vi "ma_FFT Power Spectrum and PS Density no State.vi"(0 "time signal":waveform(dbl), 1 "restart averaging (F)":bool, 2 "ps density":bool, 5 "window":T1=1 items=["Rectangle"=0, "Hanning"=1, "Hamming"=2, "Blackman-Harris"=3, "Exact Blackman"=4, "Blackman"=5, "Flat Top"=6, "4 Term B-Harris "=7, "7 Term B-Harris"=8, "Low Sidelobe"=9, "Blackman Nuttall"=11, "Triangle"=30, "Bartlett-Hanning"=31, "Bohman"=32, "Parzen"=33, "Welch"=34, "Kaiser"=60, "Dolph-Chebyshev"=61, "Gaussian"=62], 7 "averaging parameters":T3={"averaging mode"=enum."No averaging", "weighting mode"=enum."Exponential", "number of averages"=10} {"number of averages" min=1}, 9 "dB On (F)":bool, 11 "error in":errorcluster, 12 "state info":T2 {"real spectrum" format="%0.2f"; "averages completed" format="%0.2f"; "df" format="%0.2f"; "complex spectrum" format="%0.2f"; "spectrum parameters"."window" items=["Rectangle"=0, "Hanning"=1, "Hamming"=2, "Blackman-Harris"=3, "Exact Blackman"=4, "Blackman"=5, "Flat Top"=6, "4 Term B-Harris "=7, "7 Term B-Harris"=8, "Low Sidelobe"=9, "Blackman Nuttall"=11, "Triangle"=30, "Bartlett-Hanning"=31, "Bohman"=32, "Parzen"=33, "Welch"=34, "Kaiser"=60, "Dolph-Chebyshev"=61, "Gaussian"=62]; "dt" format="%0.2f"; "timestamp" format="%0.2f"; "dt history" format="%0.2f"; "t0 history" format="%0.2f"}, 13 "window parameter":dbl=nan) -> (3 "averaging done":bool, 4 "power spectrum":cluster{"f0":dbl, "df":dbl, "magnitude":dbl[]} {"f0" format="%0.2p"; "df" format="%0.2p"; "magnitude" format="%0.2p"}, 10 "averages completed":dbl format="%0.2f", 14 "state info":T2 {"real spectrum" format="%0.2f"; "averages completed" format="%0.2f"; "df" format="%0.2f"; "complex spectrum" format="%0.2f"; "spectrum parameters"."window" items=["Rectangle"=0, "Hanning"=1, "Hamming"=2, "Blackman-Harris"=3, "Exact Blackman"=4, "Blackman"=5, "Flat Top"=6, "4 Term B-Harris "=7, "7 Term B-Harris"=8, "Low Sidelobe"=9, "Blackman Nuttall"=11, "Triangle"=30, "Bartlett-Hanning"=31, "Bohman"=32, "Parzen"=33, "Welch"=34, "Kaiser"=60, "Dolph-Chebyshev"=61, "Gaussian"=62]; "dt" format="%0.2f"; "timestamp" format="%0.2f"; "dt history" format="%0.2f"; "t0 history" format="%0.2f"}, 15 "error out":errorcluster)   [LabVIEW 2020, in "NI_MAPro.lvlib"]
doc: "Computes the averaged auto power spectrum of the input signal. Each time waveform corresponds to a single FFT block and has to be passed individually to this VI. Averaging parameters specifies how the averaging is performed. This includes the averaging mode (No averaging, vector averaging, RMS averaging, or peak hold), the weighting mode (linear or exponential), and the number of averages. Averages completed returns the number of averages completed so far."
uses:
  NI_MAPro.lvlib
  windowTd.ctl
  NI_MABase.lvlib
  NI_AALPro.lvlib
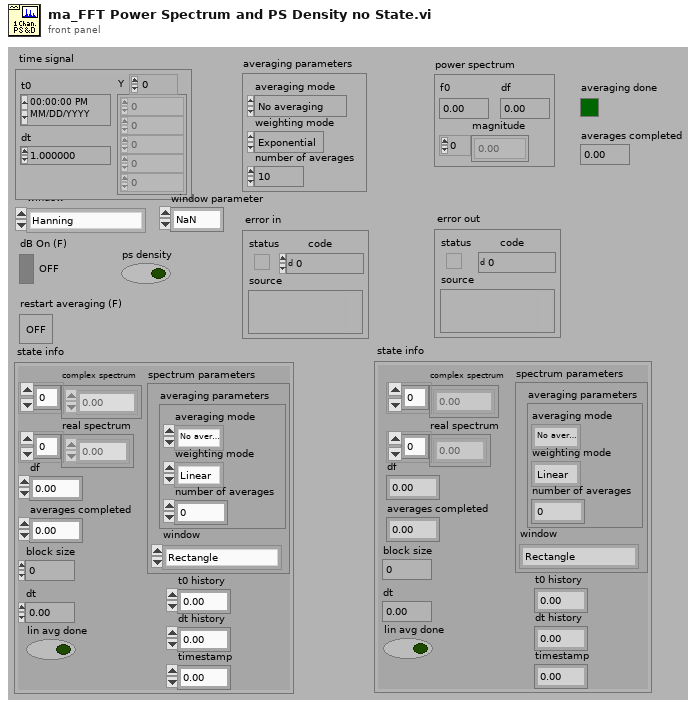
[diagram p1: front panel]
types:
  T1 = typedef "NI_AALPro.lvlib/windowTd.ctl" = u32
  T2 = cluster{"block size":i32, "dt":dbl, "spectrum parameters":cluster{"averaging parameters":cluster{"averaging mode":enum16{"No averaging", "Vector averaging", "RMS averaging", "Peak hold"}, "weighting mode":enum16{"Linear", "Exponential"}, "number of averages":u32}, "window":T1}, "df":dbl, "averages completed":dbl, "complex spectrum":cdb[], "real spectrum":dbl[], "t0 history":dbl, "dt history":dbl, "timestamp":dbl, "lin avg done":bool}
  T3 = cluster{"averaging mode":enum16{"No averaging", "Vector averaging", "RMS averaging", "Peak hold"}, "weighting mode":enum16{"Linear", "Exponential"}, "number of averages":u32}
  T4 = enum16{"FFT spectrum", "Power spectrum", "Cross spectrum", "Frequency response"}
  T5 = enum16{"No averaging", "Vector averaging", "RMS averaging", "Peak hold"}
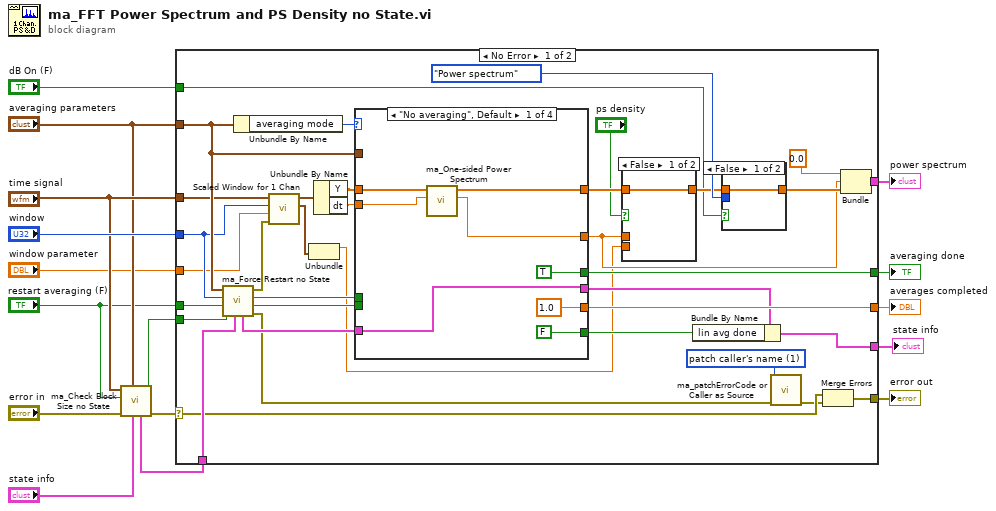
[diagram p0: block diagram]
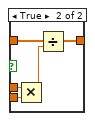
[diagram p2: hidden frame]
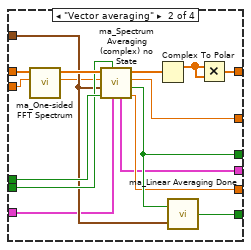
[diagram p3: hidden frame]
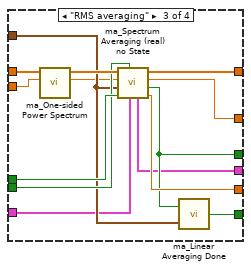
[diagram p4: hidden frame]
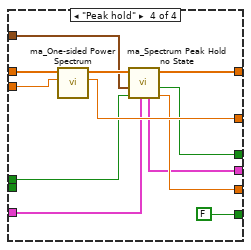
[diagram p5: hidden frame]
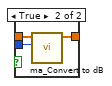
[diagram p6: hidden frame]
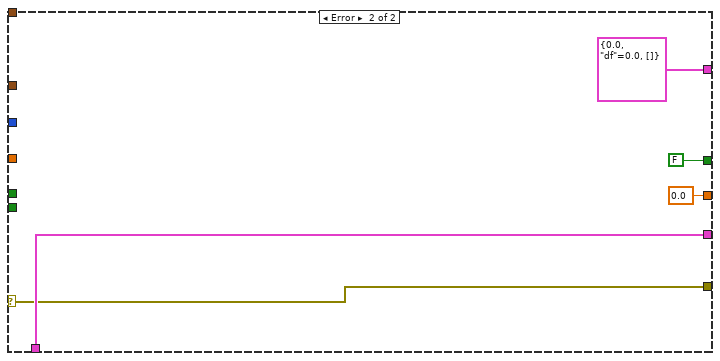
[diagram p7: hidden frame]
diagram:
  n1 = call "ma_Check Block Size no State.vi"("state info"="state info", "averaging parameters"="averaging parameters", "error in"="error in", "restart averaging (F)"="restart averaging (F)", "time signal"="time signal") -> ("error out"=w2:errorcluster, "force restart averaging"=w4:bool, "state info"=w6:T2)  [unwired: 1 in, 3 out]
  n2 = case shown="No Error" w2 {
    selector: w2 -> [w18 w113]
    tunnel: "averaging parameters" -> [w52 _]
    tunnel: [w51 0.0] -> w16
    tunnel: "window" -> [w50 _]
    tunnel: [w48 FALSE ("averaging done")] -> w14
    tunnel: "time signal" -> [w47 _]
    tunnel: "restart averaging (F)" -> [w46 _]
    tunnel: [w19 w113] -> w12
    tunnel: "dB On (F)" -> [w24 _]
    tunnel: [w43 cluster{dbl, "df":dbl, dbl[]} {0.0, "df"=0.0, []}] -> w8
    tunnel: w6 -> [w32 w114]
    tunnel: [w41 w114] -> w5
    tunnel: w4 -> [w25 _]
    tunnel: "window parameter" -> [w21 _]
    frame No Error {
      w22 = u16 1 items=["patch error code", "patch caller's name"] ("operation")
      n3 = call "ma_Force Restart no State.vi"("state info"=w32, "force restart averaging in"=w25, "restart averaging (F)"=w46, "window"=w50, "averaging parameters"=w52) -> ("error out"=w20:errorcluster, "retrieve last spectrum"=w34:bool, "force restart averaging"=w35:bool, "skip processing"=w36:errorcluster, "state info"=w33:T2)  [unwired: 1 in, 1 out]
      n4 = Unbundle By Name(w52) -> ("averaging mode"=w40:T5)
      n5 = call "Scaled Window for 1 Chan.vi"("error in (no error)"=w36, "window parameter"=w21, "window"=w50, "signal in"=w47) -> ("window constants"=w30:cluster{"eq noise BW":dbl, "coherent gain":dbl}, "signal out"=w37:waveform(dbl))  [unwired: 5 in, 1 out]
      n6 = Unbundle(w30) -> ("eq noise BW"=w23:dbl)  [unwired: 1 out]
      n7 = Unbundle By Name(w37) -> ("Y"=w38:dbl[], "dt"=w39:dbl)
      n8 = case shown="\"No averaging\", Default" w40 {
        tunnel: w38 -> [w65 w78 w94 w108]
        tunnel: [w63 w71 w88 w106] -> w27
        tunnel: [w62 w79 w95 w103] -> w29
        tunnel: w52 -> [_ w73 w89 w99]
        tunnel: w35 -> [_ w82 w96 w104]
        tunnel: [1.0 ("averages completed") w69 w86 w102] -> w51
        tunnel: w39 -> [w64 w77 w93 w107]
        tunnel: [TRUE ("averaging done") w70 w85 w100] -> w48
        tunnel: [FALSE w75 w91 FALSE] -> w42
        tunnel: w34 -> [_ w74 w90 _]
        tunnel: w33 -> [w59 w68 w84 w98]
        tunnel: [w59 w67 w83 w97] -> w31
        frame "No averaging", Default {
          n9 = call "ma_One-sided Power Spectrum.vi"("dt"=w64, "signal (V)"=w65) -> ("df"=w63:dbl, "power spectrum (V^2 rms)"=w62:dbl[])  [unwired: 1 in, 7 out]
        }
        frame "Vector averaging" {
          n10 = call "ma_One-sided FFT Spectrum.vi"("dt"=w77, "signal (V)"=w78) -> ("df"=w72:dbl, "FFT spectrum (Vrms)"=w76:cdb[])  [unwired: 1 in, 7 out]
          n11 = call "ma_Spectrum Averaging (complex) no State.vi"("state info"=w68, "retrieve last spectrum (F)"=w74, "restart averaging (F)"=w82, "averaging parameters"=w73, "df"=w72, "complex spectrum"=w76) -> ("averages completed"=w69:dbl, "averaging done"=w70:bool, "df"=w71:dbl, "averaged complex spectrum"=w81:cdb[], "state info"=w67:T2)  [unwired: 1 out]
          n12 = Complex To Polar(r * e^(i*theta)=w81) -> (r=w80:dbl[])  [unwired: 1 out]
          n13 = call "ma_Linear Averaging Done.vi"("averaging parameters"=w73, "averaging done"=w70) -> ("linear averaging done"=w75:bool)
          n14 = Multiply(x=w80, y=w80) -> (x*y=w79:dbl[])
        }
        frame "RMS averaging" {
          n15 = call "ma_One-sided Power Spectrum.vi"("dt"=w93, "signal (V)"=w94) -> ("df"=w87:dbl, "power spectrum (V^2 rms)"=w92:dbl[])  [unwired: 1 in, 7 out]
          n16 = call "ma_Spectrum Averaging (real) no State.vi"("state info"=w84, "retrieve last spectrum (F)"=w90, "restart averaging (F)"=w96, "averaging parameters"=w89, "df"=w87, "real spectrum"=w92) -> ("averages completed"=w86:dbl, "averaging done"=w85:bool, "df"=w88:dbl, "averaged real spectrum"=w95:dbl[], "state info"=w83:T2)  [unwired: 1 out]
          n17 = call "ma_Linear Averaging Done.vi"("averaging parameters"=w89, "averaging done"=w85) -> ("linear averaging done"=w91:bool)
        }
        frame "Peak hold" {
          n18 = call "ma_One-sided Power Spectrum.vi"("dt"=w107, "signal (V)"=w108) -> ("df"=w106:dbl, "power spectrum (V^2 rms)"=w105:dbl[])  [unwired: 1 in, 7 out]
          n19 = call "ma_Spectrum Peak Hold no State.vi"("state info"=w98, "restart averaging (F)"=w104, "averaging parameters"=w99, "real spectrum"=w105) -> ("averages completed"=w102:dbl, "averaging done"=w100:bool, "peak spectrum"=w103:dbl[], "state info"=w97:T2)  [unwired: 4 out]
        }
      }
      n20 = case shown="False" "ps density" {
        tunnel: w29 -> [w53 w57]
        tunnel: [w53 w56] -> w28
        tunnel: w23 -> [_ w55]
        tunnel: w27 -> [_ w54]
        frame False {
        }
        frame True {
          n21 = Multiply(x=w54, y=w55) -> (x*y=w58:dbl)
          n22 = Divide(x=w57, y=w58) -> (x/y=w56:dbl[])
        }
      }
      n23 = Bundle By Name(cluster=w31, "lin avg done"=w42) -> (w41:T2)
      n24 = case shown="False" w24 {
        tunnel: w28 -> [w109 w112]
        tunnel: [w109 w111] -> w44
        tunnel: T4."Power spectrum" ("spectrum type") -> [_ w110]
        frame False {
        }
        frame True {
          n25 = call "ma_Convert to dB.vi"("spectrum type"=w110, "spectrum"=w112) -> ("spectrum in dB"=w111:dbl[])  [unwired: 9 out]
        }
      }
      n26 = call "ma_patchErrorCode or Caller as Source.vi"("error in (no error)"=w20, "operation"=w22) -> ("error out"=w17:errorcluster)  [unwired: 2 in, 7 out]
      n27 = Merge Errors(w18, w17) -> (w19:errorcluster)
      n28 = Bundle(0.0, "df"=w27, "spectrum in dB"=w44) -> (w43:cluster{dbl, "df":dbl, "spectrum in dB":dbl[]})  [unwired: 1 out]
    }
    frame Error {
    }
  }
  "averages completed" <- w16
  "error out" <- w12
  "averaging done" <- w14
  "power spectrum" <- w8
  "state info" <- w5
